vi "ouput-plot-ple.vi"(3 "Input Cluster":T2, 4 "Data Array":i32[](array[numeric]), 5 "Wavelength Array":sgl[](array[numeric])) -> (0 "Intensity Graph":i32[][](graph), 1 "Cluster with Scaling Information":T1, 2 "Current Central Wavelength":i32)   [LabVIEW 2015]
panel:
  out "Appended Data Array":i32[][](array[numeric])
  in  "pen":T3={"Width"=1, "Style"=enum."Solid"}
  in  "color":u32(colorbox)=8978944
  in  "color table":u32[](array[colorbox])=[255, 1275, 2295, 3315, 4335, 5355, 6375, 7395, 8415, 9435, 10455, 11475, 12495, 13515, 14535, 15555, 16575, 17595, 18615, 19635, 20655, 21675, 22695, 23715, 24735, 25755, 26775, 27795, 28815, 29835, 30855, 31875, 32896, 33660, 34680, 35700, 36720, 37740, 38760, 39780, 40800, 41820, 42840, 43860, 44880, 45900, 46920, 47940, 48960, 49980, 51000, 52020, 53040, 54060, 55080, 56100, 57120, 58140, 59160, 60180, 61200, 62220, 63240, 64260, 65280, 327424, 589568, 851712, 1113856, 1376000, 1638144, 1900288, 2162432, 2424576, 2686720, 2948864, 3211008, 3473152, 3735296, 3997440, 4259584, 4521728, 4783872, 5046016, 5308160, 5570304, 5832448, 6094592, 6356736, 6618880, 6881024, 7143168, 7405312, 7667456, 7929600, 8191744, 8453888, 8650496, 8912640, 9174784, 9436928, 9699072, 9961216, 10223360, 10485504, 10747648, 11009792, 11271936, 11534080, 11796224, 12058368, 12320512, 12582656, 12844800, 13106944, 13369088, 13631232, 13893376, 14155520, 14417664, 14679808, 14941952, 15204096, 15466240, 15728384, 15990528, 16252672, 16514816, 16776960, 16776448, 16775936, 16775424, 16774912, 16774400, 16773888, 16773376, 16772864, 16772352, 16771840, 16771328, 16770816, 16770304, 16769792, 16769280, 16768768, 16768256, 16767744, 16767232, 16766720, 16766208, 16765696, 16765184, 16764672, 16764160, 16763648, 16763136, 16762624, 16762112, 16761600, 16761088, 16760832, 16760320, 16759808, 16759296, 16758784, 16758272, 16757760, 16757248, 16756736, 16756224, 16755712, 16755200, 16754688, 16754176, 16753664, 16753152, 16752640, 16752128, 16751616, 16751104, 16750592, 16750080, 16749568, 16749056, 16748544, 16748032, 16747520, 16747008, 16746496, 16745984, 16745472, 16744960, 16744448, 16743936, 16743424, 16742912, 16742400, 16741888, 16741376, 16740864, 16740352, 16739840, 16739328, 16738816, 16738304, 16737792, 16737280, 16736768, 16736256, 16735744, 16735232, 16734720, 16734208, 16733696, 16733184, 16732672, 16732160, 16731648, 16731136, 16730624, 16730112, 16729600, 16729088, 16728576, 16728064, 16727552, 16727040, 16726528, 16726016, 16725504, 16724992, 16724480, 16723968, 16723456, 16722944, 16722432, 16721920, 16721408, 16720896, 16720384, 16719872, 16719360, 16718848, 16718336, 16717824, 16717312, 16716800, 16716288, 16715776, 16715264, 16714752, 16714240, 16713728, 16713216, 16712704, 16712192]
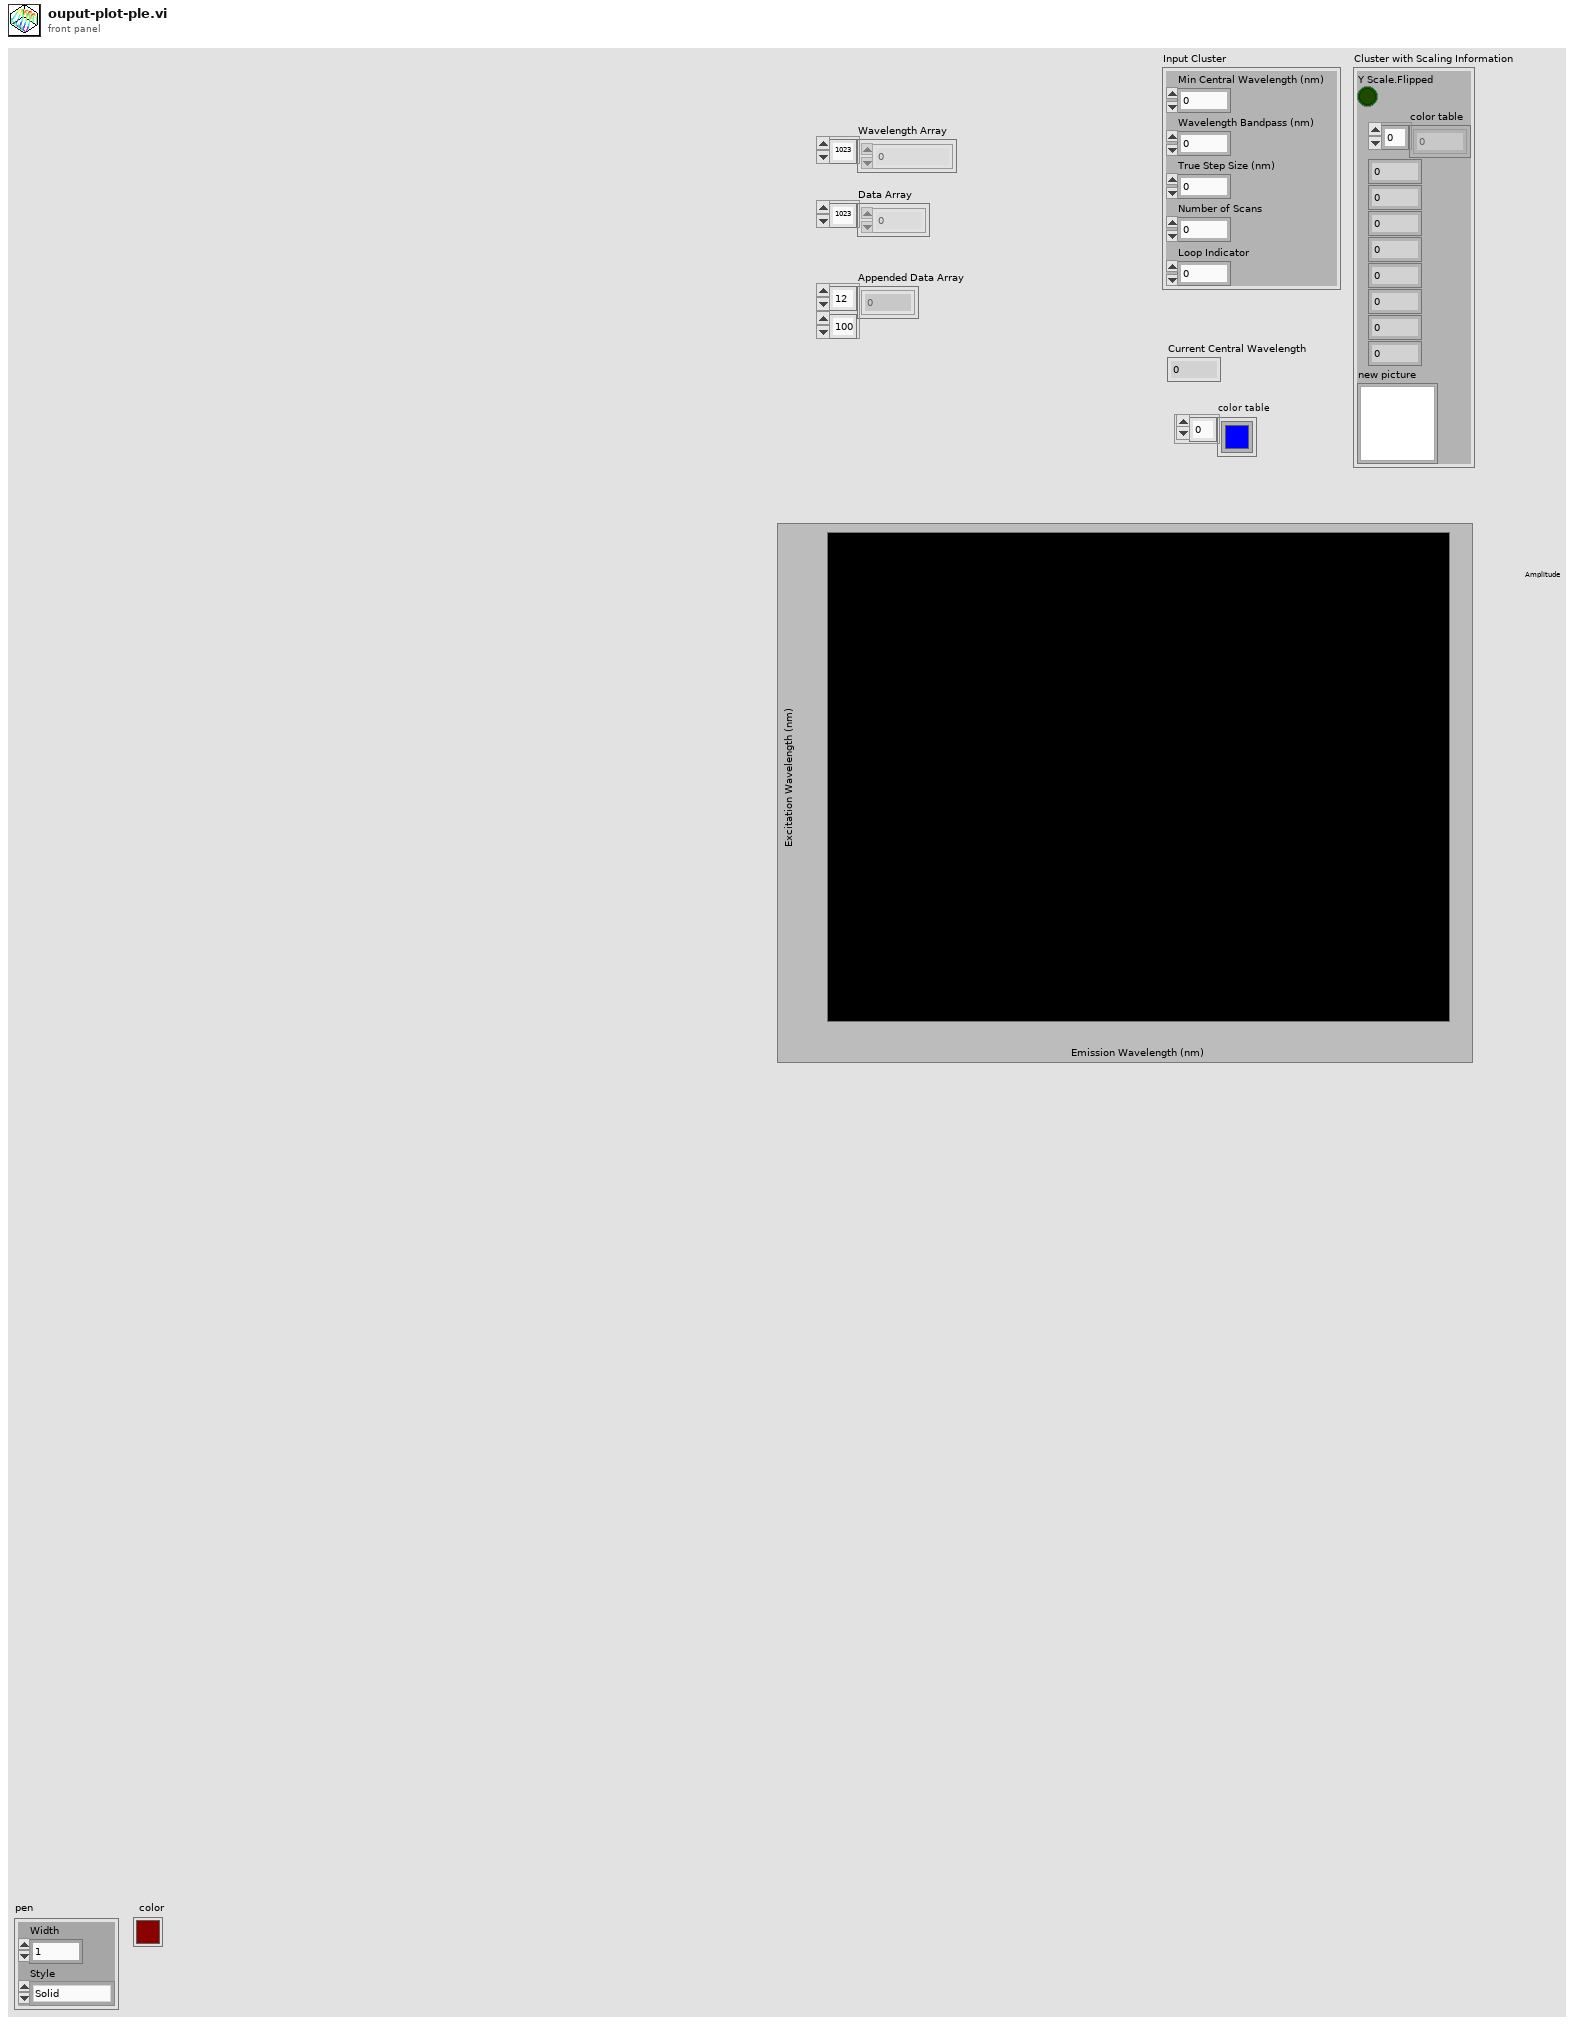
[diagram p1: front panel]
types:
  T1 = cluster{"Y Scale.Flipped":bool, "color table":u32[], dbl, dbl, dbl, dbl, sgl, sgl, sgl, dbl, "new picture":picture}
  T2 = cluster{"Min Central Wavelength (nm)":i32, "Wavelength Bandpass (nm)":i32, "True Step Size (nm) ":i32, "Number of Scans":i32, "Loop Indicator":i32}
  T3 = cluster{"Width":u16, "Style":enum32{"Solid", "Dash", "Dot", "DashDot", "DashDotDot"}}
  T4 = typedef "LVRectTypeDef.ctl" = cluster{"Left":i16, "Top":i16, "Right":i16, "Bottom":i16}
  T5 = cluster{"Y Scale.Flipped":bool, "color table":u32[], dbl, dbl, dbl, dbl, sgl, sgl, sgl, dbl}
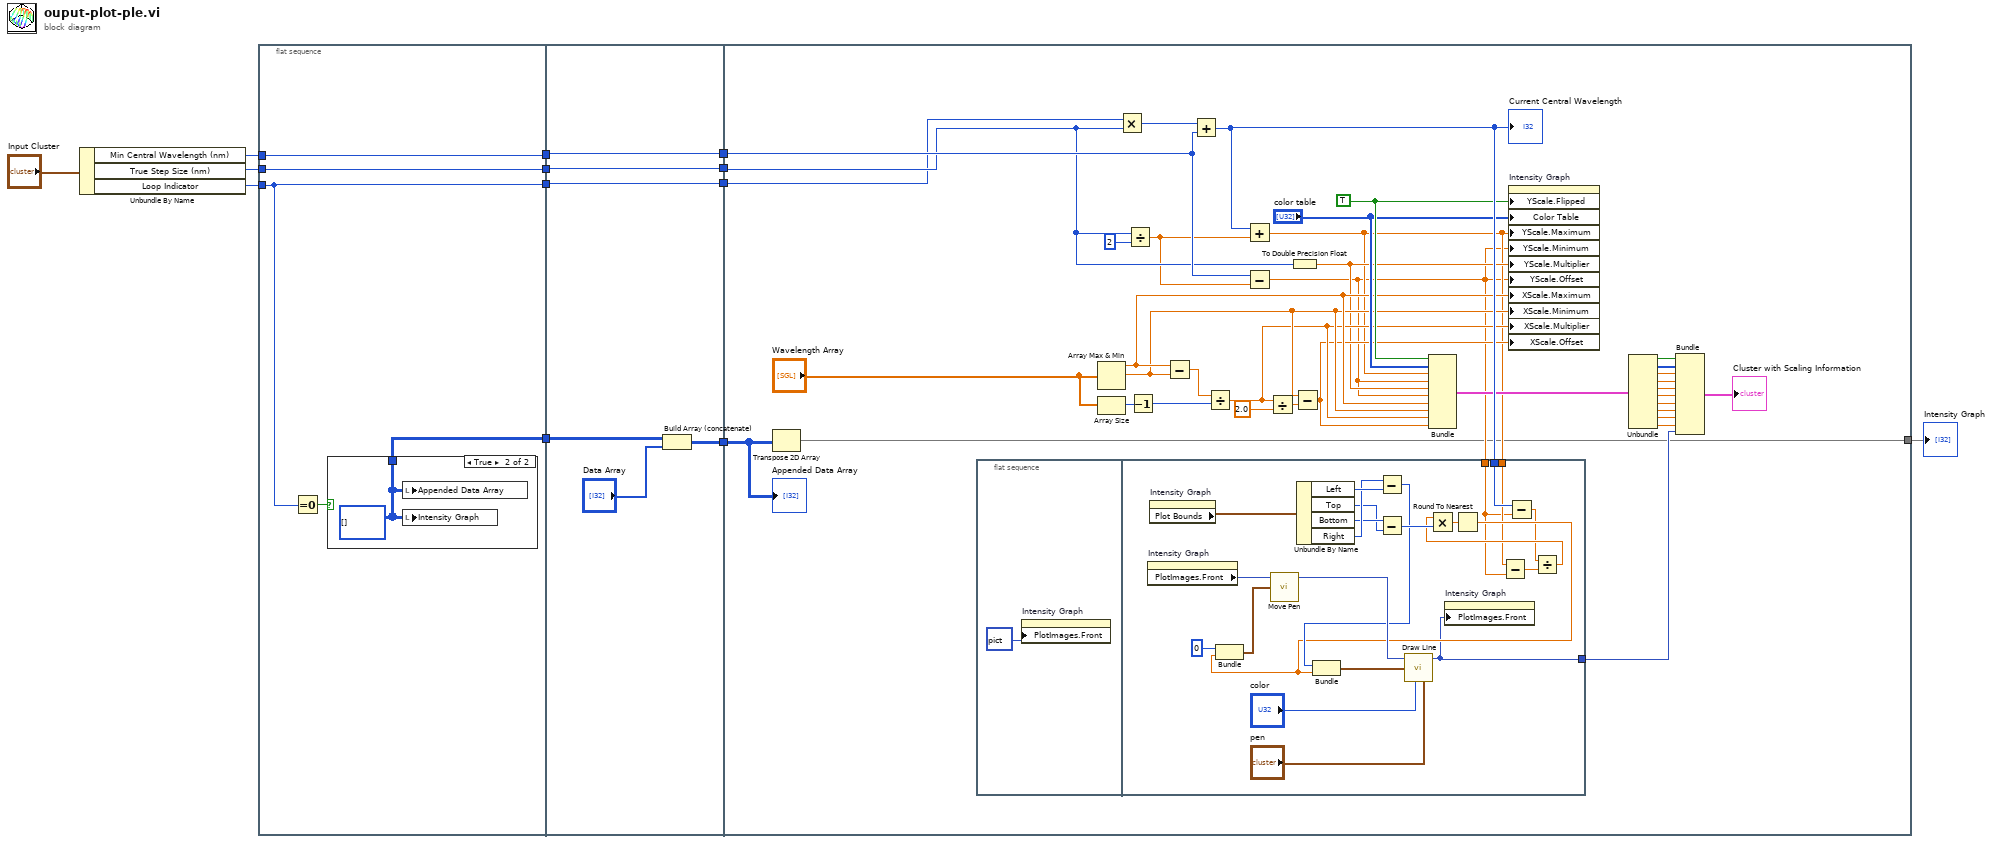
[diagram p0: block diagram]
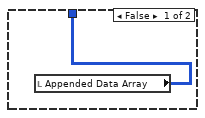
[diagram p2: hidden frame]
diagram:
  n1 = Unbundle By Name("Input Cluster") -> ("Min Central Wavelength (nm)"=w3:i32, "True Step Size (nm)"=w1:i32, "Loop Indicator"=w2:i32)
  n2 = flat-sequence {
    tunnel: [w18] -> w9
    tunnel: [w16] -> w8
    tunnel: [w14] -> w7
    tunnel: [w15] -> w6
    tunnel: w3 -> [w16]
    tunnel: w2 -> [w15]
    tunnel: w1 -> [w14]
    tunnel: [w23] -> w13
    tunnel: [w22] -> w12
    tunnel: [w21] -> w11
    tunnel: [w25] -> w10
    tunnel: w9 -> [w24]
    tunnel: w8 -> [w23]
    tunnel: w7 -> [w22]
    tunnel: w6 -> [w21]
    tunnel: w13 -> [w48]
    tunnel: w12 -> [w47]
    tunnel: w11 -> [w46]
    tunnel: w10 -> [w28]
    tunnel: [w27] -> w5
    frame #0 {
      n3 = Equal To 0?(x=w15) -> (x = 0?=w17:bool)
      n4 = case shown="True" w17 {
        tunnel: [w19 w20] -> w18
        frame False {
          n5 = local read "Appended Data Array"() -> (w19:i32[][])
        }
        frame True {
          w20 = i32[][] []
          n6 = local write "Appended Data Array"(w20) -> ()
          n7 = local write "Intensity Graph"(w20) -> ()
        }
      }
    }
    frame #1 {
      n8 = Build Array (concatenate)(w24, "Data Array") -> (w25:i32[][])
    }
    frame #2 {
      w37 = TRUE ("Y Scale.Flipped")
      n9 = Transpose 2D Array(2D array=w28) -> (transposed array=w27:i32[][])
      n10 = flat-sequence {
        tunnel: w63 -> [w68]
        tunnel: [w67] -> w50
        tunnel: w30 -> [w66]
        tunnel: w29 -> [w65]
        frame #0 {
          n11 = property on="Intensity Graph" class="IntGraph (strict)"("PlotImages.Front"=picture data[5B] ("Plot Images:Front")) -> ()  [unwired: 2 in, 2 out]
        }
        frame #1 {
          n12 = property on="Intensity Graph" class="IntGraph (strict)"() -> ("PlotImages.Front"=w85:picture)  [unwired: 2 in, 2 out]
          n13 = property on="Intensity Graph" class="IntGraph (strict)"() -> ("Plot Bounds"=w80:T4)  [unwired: 2 in, 2 out]
          n14 = Unbundle By Name(w80) -> ("Left"=w82:i16, "Top"=w77:i16, "Bottom"=w78:i16, "Right"=w81:i16)
          n15 = Subtract(x=w81, y=w82) -> (x-y=w73:i16)
          n16 = Subtract(x=w78, y=w77) -> (x-y=w75:i16)
          n17 = Subtract(x=w66, y=w65) -> (x-y=w79:dbl)
          n18 = Subtract(x=w68, y=w65) -> (x-y=w69:dbl)
          n19 = Divide(x=w69, y=w79) -> (x/y=w74:dbl)
          n20 = Multiply(x=w74, y=w75) -> (x*y=w76:dbl)
          n21 = Round To Nearest(number=w76) -> (nearest integer value=w71:dbl)
          n22 = Bundle(0, w71) -> (w70:cluster{i32, dbl})  [unwired: 1 in]
          n23 = call <vilib>:"Move Pen.vi"("new position"=w70, "picture"=w85) -> ("new picture"=w87:picture)  [unwired: 3 in]
          n24 = Bundle(w73, w71) -> (w72:cluster{i16, dbl})  [unwired: 1 in]
          n25 = call <vilib>:"Draw Line.vi"("picture"=w87, "end point"=w72, "color(black)"="color", "pen"="pen") -> ("new picture"=w67:picture)  [unwired: 5 in]
          n26 = property on="Intensity Graph" class="IntGraph (strict)"("PlotImages.Front"=w67) -> ()  [unwired: 2 in, 2 out]
        }
      }
      n27 = Array Max & Min(array="Wavelength Array") -> (max value=w35:sgl, min value=w34:sgl)  [unwired: 2 out]
      n28 = Array Size(array="Wavelength Array") -> (size(s)=w39:i32)
      n29 = Multiply(x=w46, y=w47) -> (x*y=w44:i32)
      n30 = Divide(x=w47, y=2) -> (x/y=w43:dbl)
      n31 = Decrement(x=w39) -> (x-1=w38:i32)
      n32 = Subtract(x=w35, y=w34) -> (x-y=w40:sgl)
      n33 = Add(x=w44, y=w48) -> (x+y=w63:i32)
      "Current Central Wavelength" <- w63
      n34 = Divide(x=w40, y=w38) -> (x/y=w33:sgl)
      n35 = Add(x=w63, y=w43) -> (x+y=w30:dbl)
      n36 = Subtract(x=w48, y=w43) -> (x-y=w29:dbl)
      n37 = Divide(x=w33, y=2.0) -> (x/y=w42:dbl)
      n38 = To Double Precision Float(number=w47) -> (double precision float=w31:dbl)
      n39 = Subtract(x=w34, y=w42) -> (x-y=w32:dbl)
      n40 = Bundle("Y Scale.Flipped"=w37, "color table"="color table", w30, w29, w31, w29, w35, w34, w33, w32) -> (w61:T5)  [unwired: 1 in]
      n41 = property on="Intensity Graph" class="IntGraph (strict)"("YScale.Flipped"=w37, "Color Table"="color table", "YScale.Maximum"=w30, "YScale.Minimum"=w29, "YScale.Multiplier"=w31, "YScale.Offset"=w29, "XScale.Maximum"=w35, "XScale.Minimum"=w34, "XScale.Multiplier"=w33, "XScale.Offset"=w32) -> ()  [unwired: 2 in, 2 out]
      n42 = Unbundle(w61) -> ("Y Scale.Flipped"=w60:bool, "color table"=w59:u32[], w58:dbl, w57:dbl, w56:dbl, w55:dbl, w54:sgl, w53:sgl, w52:sgl, w51:dbl)
      n43 = Bundle("Y Scale.Flipped"=w60, "color table"=w59, w58, w57, w56, w55, w54, w53, w52, w51, "new picture"=w50) -> (→"Cluster with Scaling Information":T1)  [unwired: 1 in]
      "Appended Data Array" <- w28
    }
  }
  "Intensity Graph" <- w5
